vi "parse_PolynomialSegment_array.vi"(4 "error in":errorcluster, 5 "Array Size":i32=-1, 7 "msg in":string) -> (0 "error out":errorcluster, 2 "Polynomial Segment":T1(array[cluster]), 3 "msg out":string)   [LabVIEW 2018]
doc: "Parses a message into an acceleration"
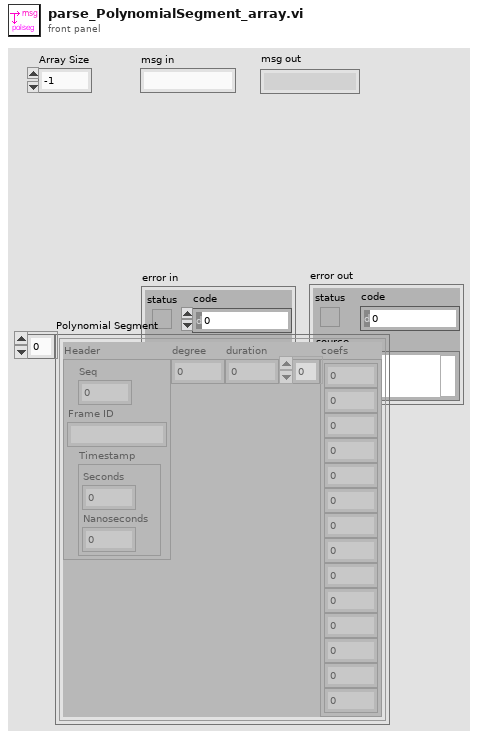
[diagram p1: front panel]
types:
  T1 = cluster{"Header":cluster{"Seq":u32, "Frame ID":string, "Timestamp":cluster{"Seconds":i32, "Nanoseconds":i32}}, "degree":i32, "duration":dbl, "coefs":dbl[]}[]
  T2 = cluster{"Header":cluster{"Seq":u32, "Frame ID":string, "Timestamp":cluster{"Seconds":i32, "Nanoseconds":i32}}, "degree":i32, "duration":dbl, "coefs":dbl[]}
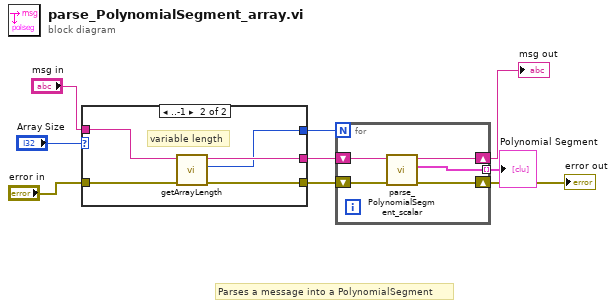
[diagram p0: block diagram]
diagram:
  # "Parses a message into a PolynomialSegment"
  n1 = case shown="..-1" "Array Size" {
    selector: "Array Size" -> [w12 _]
    tunnel: "msg in" -> [w10 w17]
    tunnel: "error in" -> [w11 w16]
    tunnel: [w12 w13] -> w6
    tunnel: [w11 w15] -> w4
    tunnel: [w10 w14] -> w5
    frame 0, Default {
      # "fixed length"
    }
    frame ..-1 {
      # "variable length"
      n2 = call "getArrayLength.vi"("error in"=w16, "msg in"=w17) -> ("error out"=w15:errorcluster, "array length"=w13:u32, "msg out"=w14:string)  [unwired: 3 in]
    }
  }
  n3 = for {
    N: w6 -> [_]
    shift-right: [w20] -> w3
    shift-left: w4 -> [w21]
    shift-right: [w19] -> w2
    shift-left: w5 -> [w22]
    tunnel: [w18] -> w1 mode=indexing
    n4 = call "parse_PolynomialSegment_scalar.vi"("error in"=w21, "msg in"=w22) -> ("error out"=w20:errorcluster, "Polynomial Segment"=w18:T2, "msg out"=w19:string)  [unwired: 3 in]
  }
  "error out" <- w3
  "msg out" <- w2
  "Polynomial Segment" <- w1
